vi "Power Switch.vi"(4 "Numeric 4":dbl, 5 "Numeric 2":dbl, 6 "Numeric 3":dbl, 7 "Numeric":dbl, 8 "Boolean 4":bool, 9 "Boolean 3":bool, 10 "Boolean 2":bool, 11 "Boolean":bool) -> (2 "Numeric Out":dbl)   [LabVIEW 2015]
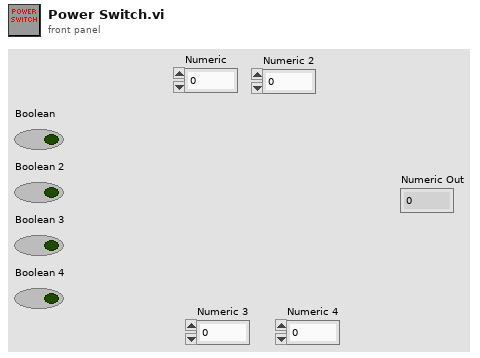
[diagram p1: front panel]
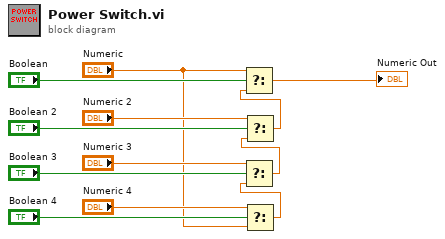
[diagram p0: block diagram]
diagram:
  n1 = Select(t="Numeric 4", s="Boolean 4", f="Numeric") -> (s? t:f=w3:dbl)
  n2 = Select(t="Numeric 3", s="Boolean 3", f=w3) -> (s? t:f=w4:dbl)
  n3 = Select(t="Numeric 2", s="Boolean 2", f=w4) -> (s? t:f=w5:dbl)
  n4 = Select(t="Numeric", s="Boolean", f=w5) -> (s? t:f=→"Numeric Out":dbl)
